vi "PC_test.vi"() -> ()   [LabVIEW 2018]
uses:
  <vilib>/express/express signal manip/GetorSetDDTAttributes/Set DDT Attributes/Set DDT Properties.xnode
  <vilib>/express/express shared/transition.llb/Dynamic To Waveform Array.vi
  <vilib>/express/express signal manip/GetorSetDDTAttributes/Set DDT Attributes/SetT0.vi
  <vilib>/express/express shared/transition.llb/Waveform Array To Dynamic.vi
  <vilib>/Analysis/NI_AALPro.lvlib
  <vilib>/Analysis/coordinate.llb/Euler Rotation Order.ctl
  <vilib>/Analysis/NI_AALBase.lvlib
  <vilib>/Analysis/Matrix/Datatypes/RealMatrix.ctl
  <vilib>/Analysis/Matrix/NI_Matrix.lvlib
  <vilib>/Analysis/coordinate.llb/3D Cartesian Coordinate Rotation (Euler) (Array).vi
  <vilib>/Analysis/coordinate.llb/3D Cartesian Coordinate Rotation (Direction) (Array).vi
  <vilib>/Analysis/baseanly.llb/Real A x B.vi
  <vilib>/Analysis/baseanly.llb/Real Outer Product.vi
  <vilib>/Analysis/Matrix/Numeric/Multiply/Multiply - RM,R.vi
  <vilib>/Analysis/Matrix/Numeric/Multiply/Multiply - R,RM.vi
panel:
  out "_LED 1":dbl[](array[numeric])
  out "_LED 2":dbl[](array[numeric])
  out "_LED3":dbl[](array[numeric])
  out "_LED4":dbl[](array[numeric])
  out "c * A":T1
  out "Outer Product":T1
  in  "A Vector 3":dbl[](array[numeric])
  in  "A Vector 2":dbl[](array[numeric])
  out "Direction Cosines 4":dbl[][](array[numeric])
  out "alpha":dbl
  out "beta":dbl
  in  "A Vector":dbl[](array[numeric])
  out "Direction Cosines 3":dbl[][](array[numeric])
  out "Euler Angles 3":cluster{"phi":dbl, "theta":dbl, "psi":dbl}
  out "Cross Product":dbl[](array[numeric])
  out "Euler Angles 2":cluster{"phi":dbl, "theta":dbl, "psi":dbl}
  out "transposed matrix":T1
  out "Direction Cosines 2":dbl[][](array[numeric])
  out "appended array":dbl[][](array[numeric])
  out "A x B":T1
  out "Direction Cosines":dbl[][](array[numeric])
  out "Euler Angles":cluster{"phi":dbl, "theta":dbl, "psi":dbl}
  out "x/y":dbl
  out "Result":dbl[][](array[numeric])
  in  "Root length":i32
  in  "Repeat inteval":dbl
  in  "Command":dbl
  in  "Repeat times":i32
  in  "Boolean":bool
  in  "array 3":dbl[][](array[numeric])
  out "v":u16
  out "Commands 2":u16(ring)=2 items=["MoveJoints"=1, "MovePose"=2, "MoveLin"=3, "MoveLinRelTRF"=4, "MoveLinRelWRF"=5]
  in  "Commands":u16(ring) items=["MoveJoints"=1, "MovePose"=2, "MoveLin"=3, "MoveLinRelTRF"=4, "MoveLinRelWRF"=5]
  out "element 3":dbl
  out "element 2":dbl
  out "element":dbl
  in  "y 3":dbl[](array[numeric])
  out "arccos(x)":dbl
  out "cos(x)":dbl
  out "spreadsheet string":string
  in  "array 2":dbl[][](array[numeric])
  out "array":dbl[][](array[numeric])
  # "Wating for activating..."
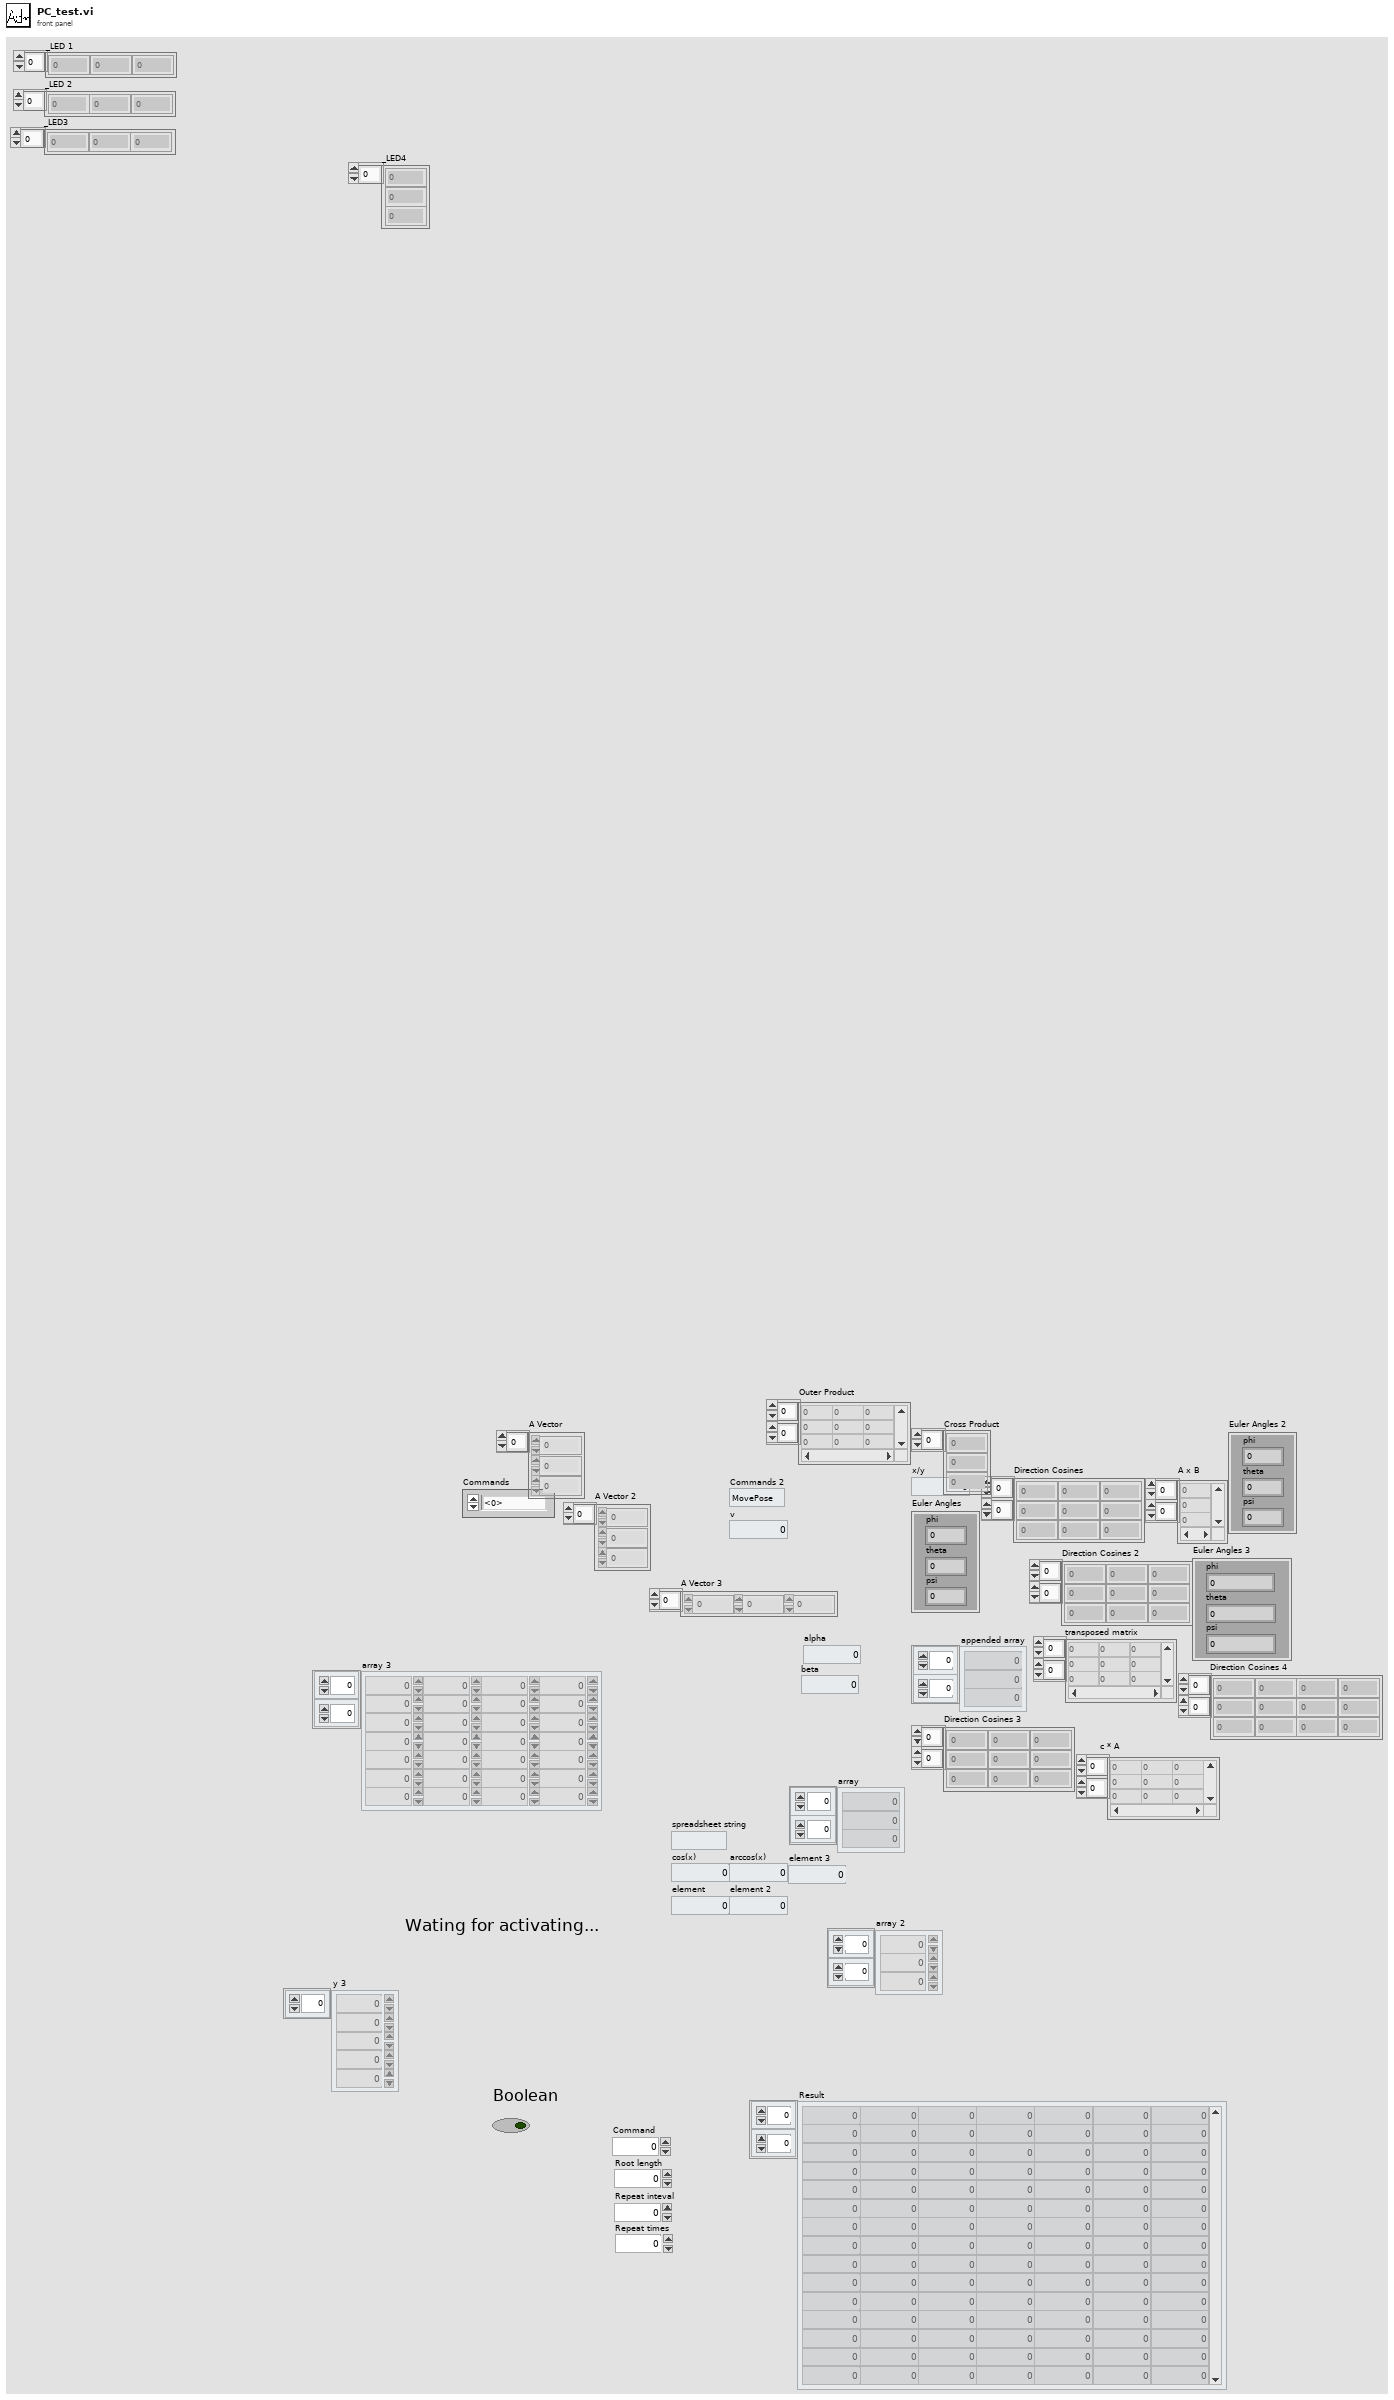
[diagram p1: front panel]
types:
  T1 = typedef "NI_Matrix.lvlib/RealMatrix.ctl" = dbl[][]
  T2 = typedef "NI_AALPro.lvlib/Euler Rotation Order.ctl" = u16
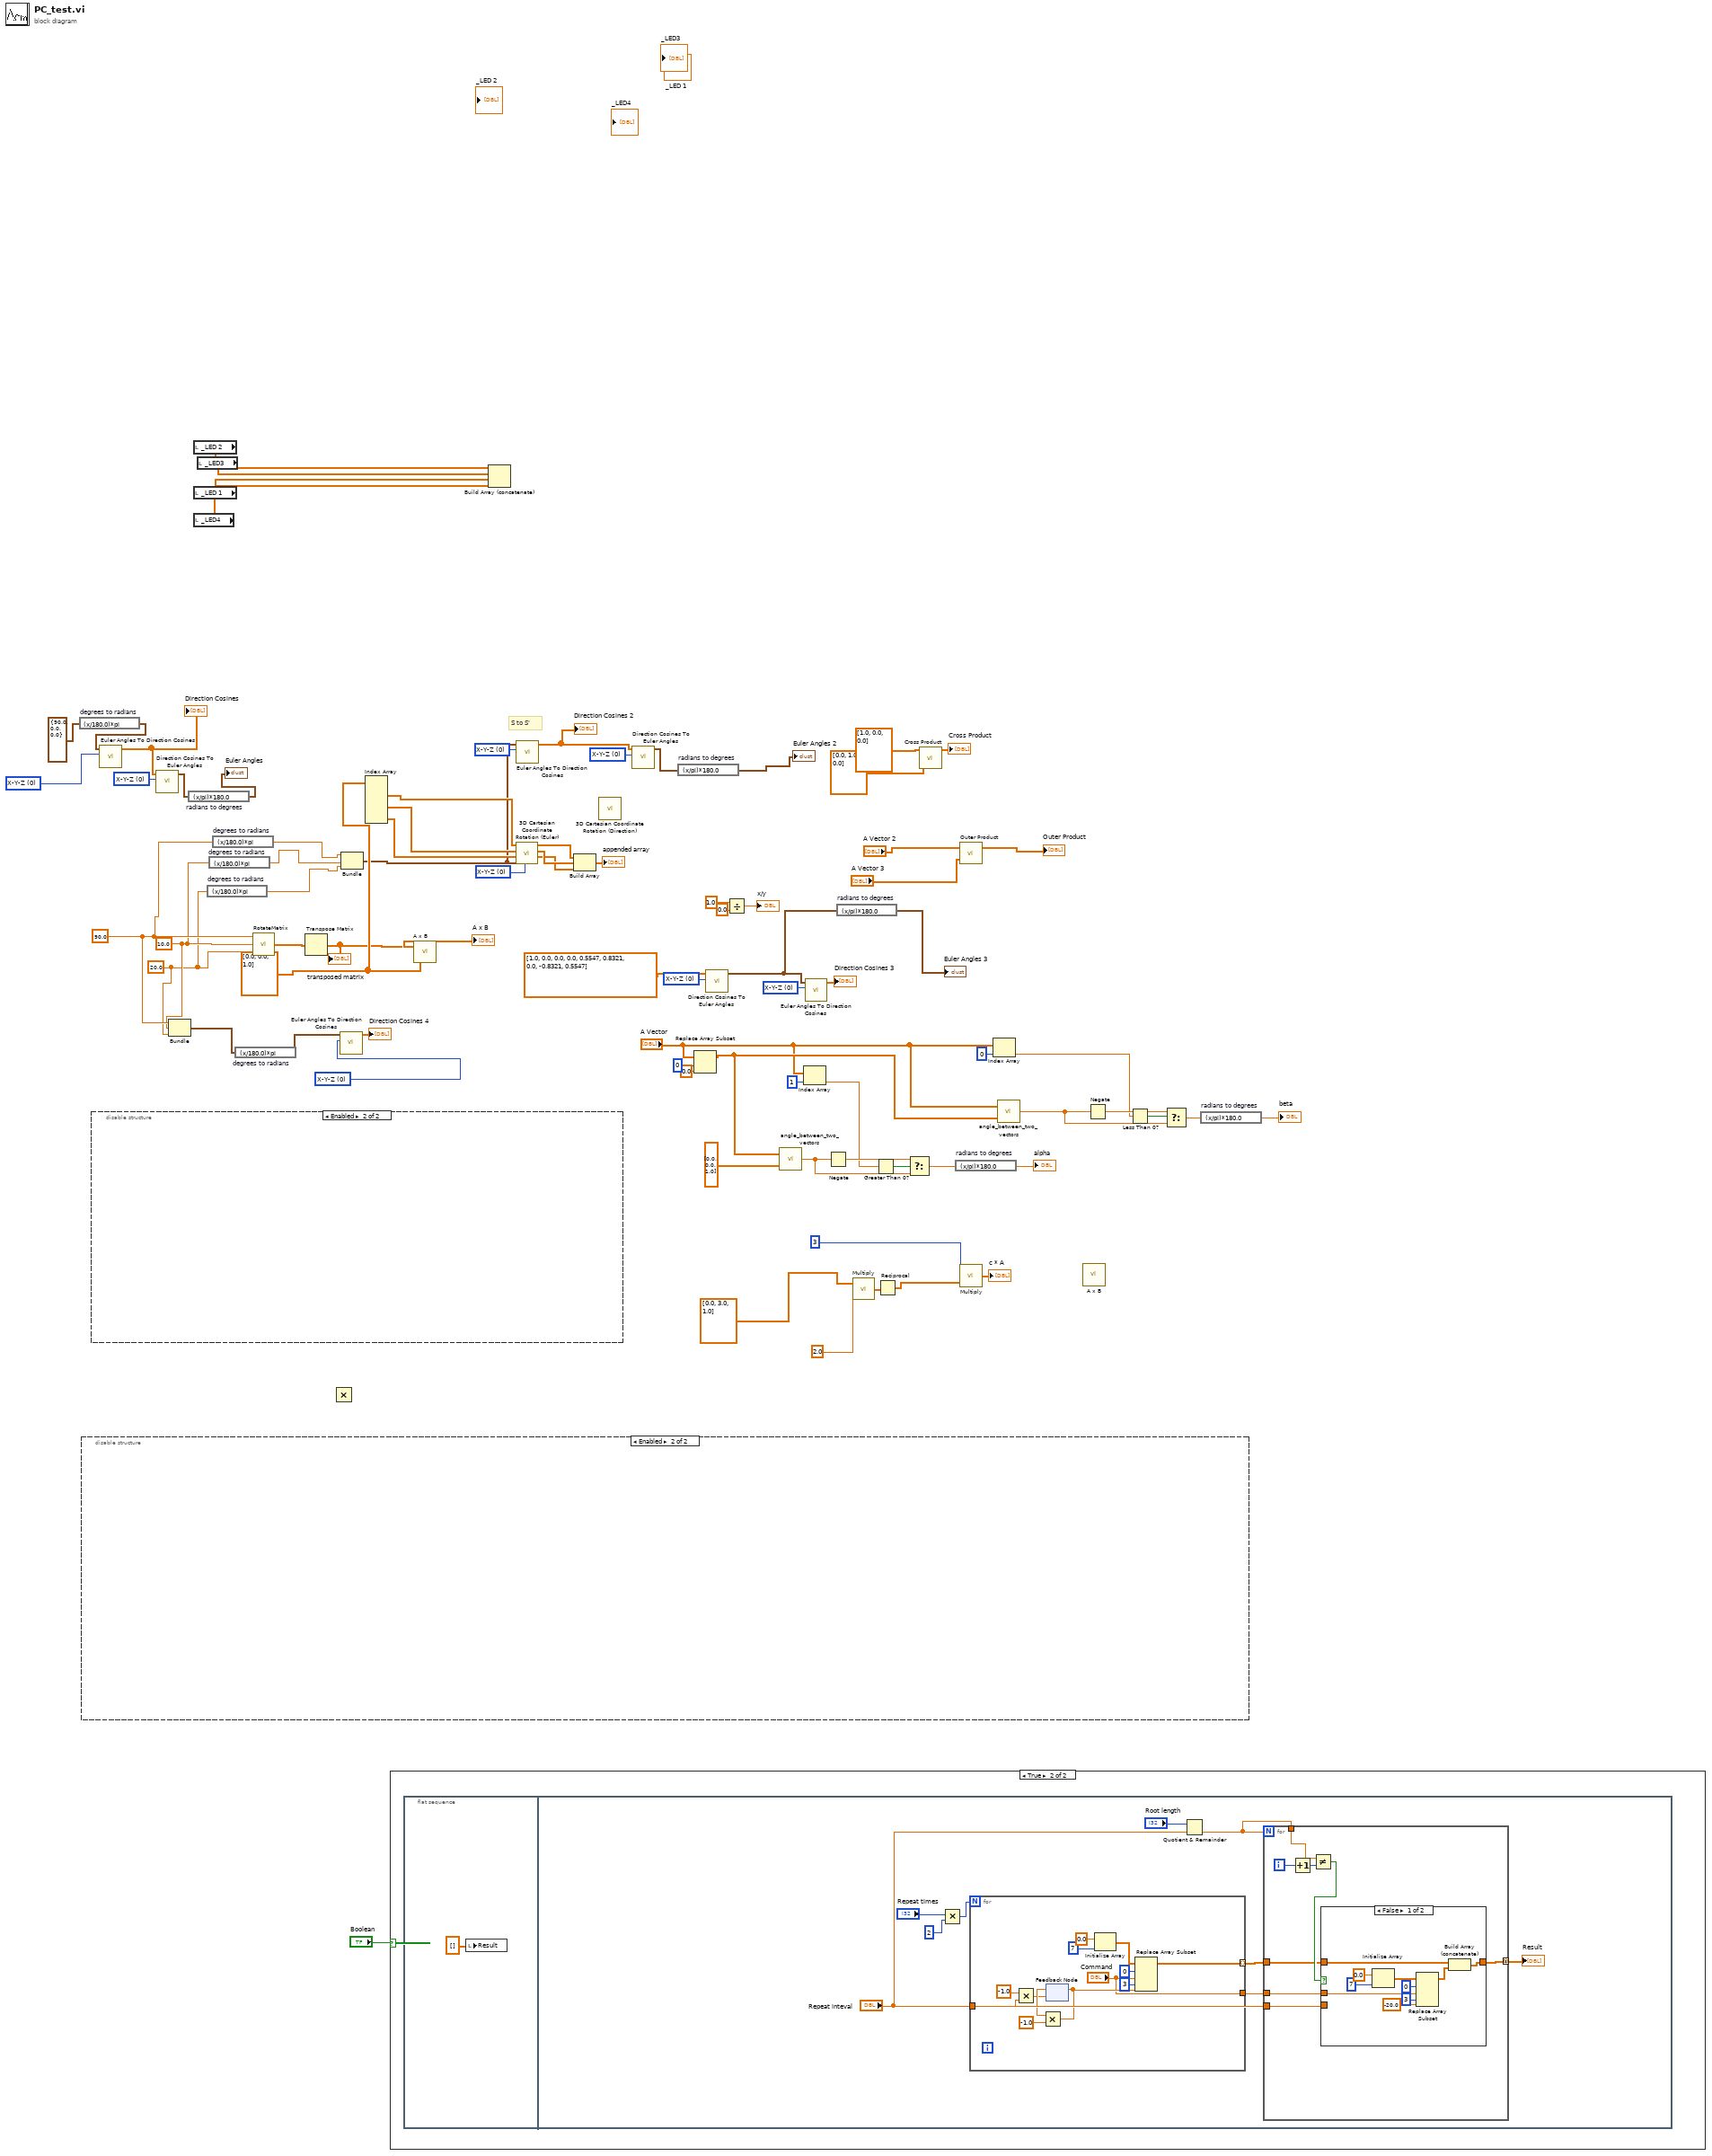
[diagram p0: block diagram]
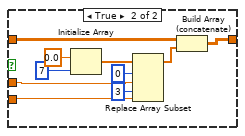
[diagram p3: hidden frame]
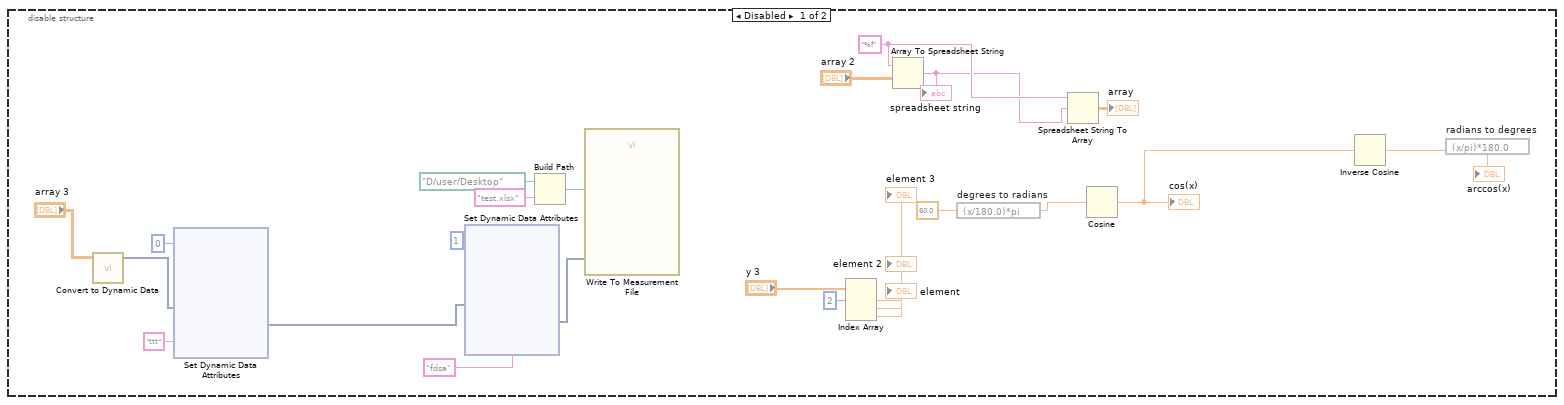
[diagram p4: hidden frame]
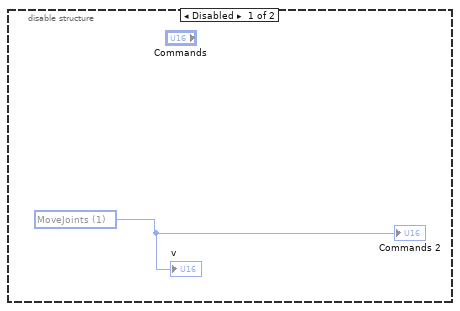
[diagram p5: hidden frame]
diagram:
  w19 = T2 0 items=["X-Y-Z", "X-Z-Y", "Y-X-Z", "Y-Z-X", "Z-X-Y", "Z-Y-X", "X-Y-X", "X-Z-X", "Y-X-Y", "Y-Z-Y", "Z-X-Z", "Z-Y-Z"] ("rotation order")
  w40 = T2 0 items=["X-Y-Z", "X-Z-Y", "Y-X-Z", "Y-Z-X", "Z-X-Y", "Z-Y-X", "X-Y-X", "X-Z-X", "Y-X-Y", "Y-Z-Y", "Z-X-Z", "Z-Y-Z"] ("rotation order")
  w44 = T2 0 items=["X-Y-Z", "X-Z-Y", "Y-X-Z", "Y-Z-X", "Z-X-Y", "Z-Y-X", "X-Y-X", "X-Z-X", "Y-X-Y", "Y-Z-Y", "Z-X-Z", "Z-Y-Z"] ("rotation order")
  w55 = T2 0 items=["X-Y-Z", "X-Z-Y", "Y-X-Z", "Y-Z-X", "Z-X-Y", "Z-Y-X", "X-Y-X", "X-Z-X", "Y-X-Y", "Y-Z-Y", "Z-X-Z", "Z-Y-Z"] ("rotation order")
  w57 = T2 0 items=["X-Y-Z", "X-Z-Y", "Y-X-Z", "Y-Z-X", "Z-X-Y", "Z-Y-X", "X-Y-X", "X-Z-X", "Y-X-Y", "Y-Z-Y", "Z-X-Z", "Z-Y-Z"] ("rotation order")
  w61 = T2 0 items=["X-Y-Z", "X-Z-Y", "Y-X-Z", "Y-Z-X", "Z-X-Y", "Z-Y-X", "X-Y-X", "X-Z-X", "Y-X-Y", "Y-Z-Y", "Z-X-Z", "Z-Y-Z"] ("rotation order")
  w69 = T1 [[0.0], [0.0], [1.0]] ("B")
  w15 = 20.0 ("gamma")
  w16 = 10.0 ("beta")
  w17 = 90.0 ("alpha")
  w74 = T2 0 items=["X-Y-Z", "X-Z-Y", "Y-X-Z", "Y-Z-X", "Z-X-Y", "Z-Y-X", "X-Y-X", "X-Z-X", "Y-X-Y", "Y-Z-Y", "Z-X-Z", "Z-Y-Z"] ("rotation order")
  w75 = T2 0 items=["X-Y-Z", "X-Z-Y", "Y-X-Z", "Y-Z-X", "Z-X-Y", "Z-Y-X", "X-Y-X", "X-Z-X", "Y-X-Y", "Y-Z-Y", "Z-X-Z", "Z-Y-Z"] ("rotation order")
  # "S to S'"
  n1 = expression code="(x/180.0)*pi" "degrees to radians"(cluster{"phi":dbl, "theta":dbl, "psi":dbl} {"phi"=90.0, "theta"=0.0, "psi"=0.0} ("Euler Angles")) -> (w49:cluster{"phi":dbl, "theta":dbl, "psi":dbl})
  n2 = disable-structure shown="Enabled" {
    frame Disabled {
      w103 = "%f" ("format string")
      n3 = call "Convert to Dynamic Data"("2D Array"="array 3") -> ("Dynamic Data Type"=w86:dynamicdata)  [unwired: 3 in]
      n4 = xnode "Set Dynamic Data Attributes"("Signals In"=w86, "Signal Name"="ttt", "Signal Index"=0) -> ("Signals Out"=w84:dynamicdata)  [unwired: 1 in, 1 out]
      n5 = xnode "Set Dynamic Data Attributes"("Signals In"=w84, "Signal Name"="fdsa", "Signal Index"=1) -> ("Signals Out"=w83:dynamicdata)  [unwired: 1 in, 1 out]
      n6 = Build Path(base path=path "D:/user/Desktop", name or relative path="test.xlsx") -> (appended path=w89:path)
      n7 = call "Write To Measurement File"("Signals"=w83, "Filename"=w89) -> ()  [unwired: 15 in, 3 out]
      n8 = Index Array(array="y 3", index #1=2 ("index")) -> (element #1=→"element":dbl, element #2=→"element 2":dbl, element #3=→"element 3":dbl)  [unwired: 2 in]
      n9 = Array To Spreadsheet String(array="array 2", 3:w103) -> (spreadsheet string=w102:string)  [unwired: 1 in]
      "spreadsheet string" <- w102
      n10 = expression code="(x/180.0)*pi" "degrees to radians"(60.0 ("x")) -> (w99:dbl)
      n11 = Spreadsheet String To Array(format string=w103, spreadsheet string=w102) -> (array=→"array":dbl[][])  [unwired: 2 in]
      n12 = Cosine(x=w99) -> (cos(x)=w101:dbl)
      "cos(x)" <- w101
      n13 = Inverse Cosine(1:w101) -> (0:w98:dbl)
      n14 = expression code="(x/pi)*180.0" "radians to degrees"(w98) -> (→"arccos(x)":dbl)
    }
    frame Enabled {
    }
  }
  n15 = disable-structure shown="Enabled" {
    frame Disabled {
      w132 = u16 1 items=["MoveJoints"=1, "MovePose"=2, "MoveLin"=3, "MoveLinRelTRF"=4, "MoveLinRelWRF"=5] ("Commands")
      "Commands 2" <- w132
      "v" <- w132
    }
    frame Enabled {
    }
  }
  n16 = call <vilib>:"Euler Angles To Direction Cosines.vi"("rotation order"=w75, "Euler Angles"=w49) -> ("Direction Cosines"=w76:dbl[][])  [unwired: 8 in, 1 out]
  "Direction Cosines" <- w76
  n17 = call <vilib>:"Direction Cosines To Euler Angles.vi"("rotation order"=w74, "Direction Cosines"=w76) -> ("Euler Angles"=w52:cluster{"phi":dbl, "theta":dbl, "psi":dbl})  [unwired: 8 in, 1 out]
  n18 = Bundle("alpha"=w17, "beta"=w16, "gamma"=w15) -> (w14:cluster{"alpha":dbl, "beta":dbl, "gamma":dbl})  [unwired: 1 in]
  n19 = expression code="(x/pi)*180.0" "radians to degrees"(w52) -> (→"Euler Angles":cluster{"phi":dbl, "theta":dbl, "psi":dbl})
  n20 = local read "_LED 2"() -> (w4:dbl[])
  n21 = local read "_LED 1"() -> (w2:dbl[])
  n22 = local read "_LED4"() -> (w1:dbl[])
  n23 = local read "_LED3"() -> (w3:dbl[])
  n24 = expression code="(x/180.0)*pi" "degrees to radians"(w15) -> (w70:dbl)
  n25 = expression code="(x/180.0)*pi" "degrees to radians"(w16) -> (w71:dbl)
  n26 = expression code="(x/180.0)*pi" "degrees to radians"(w17) -> (w72:dbl)
  n27 = expression code="(x/180.0)*pi" "degrees to radians"(w14) -> (w20:cluster{"alpha":dbl, "beta":dbl, "gamma":dbl})
  n28 = call "RotateMatrix.vi"("gamma"=w15, "beta"=w16, "alpha"=w17) -> ("Rotate Matrix"=w60:T1)
  n29 = Transpose Matrix(1:w60) -> (0:w59:T1)
  "transposed matrix" <- w59
  n30 = Multiply ("Multiply 2")() -> ()  [unwired: 2 in, 1 out]
  n31 = call <vilib>:"Euler Angles To Direction Cosines.vi"("rotation order"=w19, "Euler Angles"=w20) -> ("Direction Cosines"=→"Direction Cosines 4":dbl[][])  [unwired: 8 in, 1 out]
  n32 = Bundle("alpha"=w72, "beta"=w71, "gamma"=w70) -> (w58:cluster{"alpha":dbl, "beta":dbl, "gamma":dbl})  [unwired: 1 in]
  n33 = Index Array(array=w69) -> (element #1=w68:dbl[], element #2=w67:dbl[], element #3=w66:dbl[])  [unwired: 6 in]
  n34 = case shown="True" "Boolean" {
    frame False {
    }
    frame True {
      n35 = flat-sequence {
        frame #0 {
          n36 = local write "Result"(dbl[][] [] ("Result")) -> ()
        }
        frame #1 {
          n37 = Multiply(x="Repeat times", y=2) -> (x*y=w141:i32)
          n38 = for {
            N: w141 -> [_]
            tunnel: "Repeat inteval" -> [w146]
            tunnel: [w143] -> w135 mode=indexing
            tunnel: ["Command"] -> w138
            n39 = Multiply(x=-1.0 ("y"), y=w146) -> (x*y=w145:dbl)
            n40 = feedback #1(w145) -> (w155:dbl)
            n41 = Multiply(x=w155, y=-1.0) -> (x*y=w148:dbl)
            n42 = feedback-in #1(w148) -> ()
            n43 = Initialize Array(0.0 ("element"), 7 ("dimension size")) -> (w151:dbl[])
            n44 = Replace Array Subset(array=w151, new element #1="Command", index #1=0 ("index"), new element #2=w148, index #2=3 ("index")) -> (w143:dbl[])
          }
          n45 = Quotient & Remainder(x="Root length", y="Repeat inteval") -> (floor(x/y)=w134:dbl)  [unwired: 1 out]
          n46 = for {
            N: w134 -> [_]
            tunnel: w134 -> [w162]
            tunnel: w135 -> [w157]
            tunnel: w138 -> [w159]
            tunnel: "Repeat inteval" -> [w158]
            tunnel: [w156] -> w136 mode=concatenating
            i -> [w161]
            n47 = Increment(x=w161) -> (x+1=w163:i32)
            n48 = Not Equal?(x=w162, y=w163) -> (x != y?=w160:bool)
            n49 = case shown="False" w160 {
              tunnel: w159 -> [w166 w177]
              tunnel: w158 -> [_ w176]
              tunnel: w157 -> [w165 w175]
              tunnel: [w167 w174] -> w156
              frame False {
                n50 = Initialize Array(0.0 ("element"), 7 ("dimension size")) -> (w171:dbl[])
                n51 = Replace Array Subset(array=w171, new element #1=w166, index #1=0 ("index"), new element #2=-20.0 ("new element/subarray"), index #2=3 ("index")) -> (w168:dbl[])
                n52 = Build Array (concatenate)(w165, w168) -> (w167:dbl[][])
              }
              frame True {
                n53 = Initialize Array(0.0 ("element"), 7 ("dimension size")) -> (w181:dbl[])
                n54 = Replace Array Subset(array=w181, new element #1=w177, index #1=0 ("index"), new element #2=w176, index #2=3 ("index")) -> (w178:dbl[])
                n55 = Build Array (concatenate)(w175, w178) -> (w174:dbl[][])
              }
            }
          }
          "Result" <- w136
        }
      }
    }
  }
  n56 = call-poly <vilib>:"A x B.vi"("B"=w69, "A"=w59) -> ("A x B"=→"A x B":T1)  [unwired: 1 out]
  n57 = Build Array (concatenate)(w4, w3, w2, w1) -> ()  [unwired: 1 out]
  n58 = call-poly <vilib>:"3D Cartesian Coordinate Rotation (Euler).vi"("rotation order"=w61, "Euler Angles"=w58, "Z"=w66, "Y"=w67, "X"=w68) -> ("Z Out"=w63:dbl[], "Y Out"=w64:dbl[], "X Out"=w65:dbl[])  [unwired: 3 in, 1 out]
  n59 = call <vilib>:"Euler Angles To Direction Cosines.vi"("rotation order"=w57, "Euler Angles"=w58) -> ("Direction Cosines"=w56:dbl[][])  [unwired: 8 in, 1 out]
  "Direction Cosines 2" <- w56
  n60 = Build Array(w65, w64, w63) -> (→"appended array":dbl[][])
  n61 = call-poly <vilib>:"3D Cartesian Coordinate Rotation (Direction).vi"() -> ()  [unwired: 8 in, 4 out]
  n62 = call <vilib>:"Direction Cosines To Euler Angles.vi"("rotation order"=w55, "Direction Cosines"=w56) -> ("Euler Angles"=w54:cluster{"phi":dbl, "theta":dbl, "psi":dbl})  [unwired: 8 in, 1 out]
  n63 = expression code="(x/pi)*180.0" "radians to degrees"(w54) -> (→"Euler Angles 2":cluster{"phi":dbl, "theta":dbl, "psi":dbl})
  n64 = Replace Array Subset(array="A Vector", new element=0.0 ("new element/subarray"), index=0) -> (w34:dbl[])
  n65 = call <vilib>:"Direction Cosines To Euler Angles.vi"("rotation order"=w44, "Direction Cosines"=dbl[][] [[1.0, 0.0, 0.0], [0.0, 0.5547, 0.8321], [0.0, -0.8321, 0.5547]]) -> ("Euler Angles"=w42:cluster{"phi":dbl, "theta":dbl, "psi":dbl})  [unwired: 8 in, 1 out]
  n66 = Divide(x=1.0, y=0.0) -> (x/y=→"x/y":dbl)
  n67 = call "angle_between_two_vectors.vi"("B Vector"=dbl[] [0.0, 0.0, 1.0], "A Vector"=w34) -> ("degree"=w36:dbl)
  n68 = Index Array(array="A Vector", index=1) -> (element=w26:dbl)
  n69 = call <vilib>:"Euler Angles To Direction Cosines.vi"("rotation order"=w40, "Euler Angles"=w42) -> ("Direction Cosines"=→"Direction Cosines 3":dbl[][])  [unwired: 8 in, 1 out]
  n70 = Negate(x=w36) -> (-x=w35:dbl)
  n71 = expression code="(x/pi)*180.0" "radians to degrees"(w42) -> (→"Euler Angles 3":cluster{"phi":dbl, "theta":dbl, "psi":dbl})
  n72 = call-poly <vilib>:"Multiply.vi"("Real Scalar c"=2.0 ("Numeric"), "Real Matrix A"=T1 [[0.0], [3.0], [1.0]] ("B")) -> ("A * c"=w8:T1)
  n73 = Greater Than 0?(x=w26) -> (x > 0?=w25:bool)
  n74 = Reciprocal(x=w8) -> (1/x=w6:T1)
  n75 = Select(t=w35, s=w25, f=w36) -> (s? t:f=w29:dbl)
  n76 = call <vilib>:"Cross Product.vi"("B Vector"=dbl[] [0.0, 1.0, 0.0], "A Vector"=dbl[] [1.0, 0.0, 0.0]) -> ("Cross Product"=→"Cross Product":dbl[])  [unwired: 8 in, 1 out]
  n77 = expression code="(x/pi)*180.0" "radians to degrees"(w29) -> (→"alpha":dbl)
  n78 = call-poly <vilib>:"Outer Product.vi"("Y Vector"="A Vector 3", "X Vector"="A Vector 2") -> ("Outer Product"=→"Outer Product":T1)  [unwired: 1 out]
  n79 = call-poly <vilib>:"Multiply.vi"("Real Matrix A"=w6, "Real Scalar c"=3 ("Numeric")) -> ("c * A"=→"c * A":T1)
  n80 = Index Array(array="A Vector", index=0) -> (element=w22:dbl)
  n81 = call "angle_between_two_vectors.vi"("B Vector"=w34, "A Vector"="A Vector") -> ("degree"=w33:dbl)
  n82 = call-poly <vilib>:"A x B.vi"() -> ()  [unwired: 2 in, 2 out]
  n83 = Negate(x=w33) -> (-x=w30:dbl)
  n84 = Less Than 0?(x=w22) -> (x < 0?=w21:bool)
  n85 = Select(t=w30, s=w21, f=w33) -> (s? t:f=w32:dbl)
  n86 = expression code="(x/pi)*180.0" "radians to degrees"(w32) -> (→"beta":dbl)
